vi "Check CSM Modules Exist Or Not.vi"(8 "error in":errorcluster, 11 "CSM names in":string[](array[string])) -> (0 "error out":errorcluster, 2 "Debug string":string, 3 "All Modules Exist?":bool)   [LabVIEW 2017]
uses:
  src/user.lib/_NEVSTOP/Communicable State Machine(CSM)/Communicable State Machine.lvlib
  src/user.lib/_NEVSTOP/Communicable State Machine(CSM)/_Shared/CSM Shared.lvlib
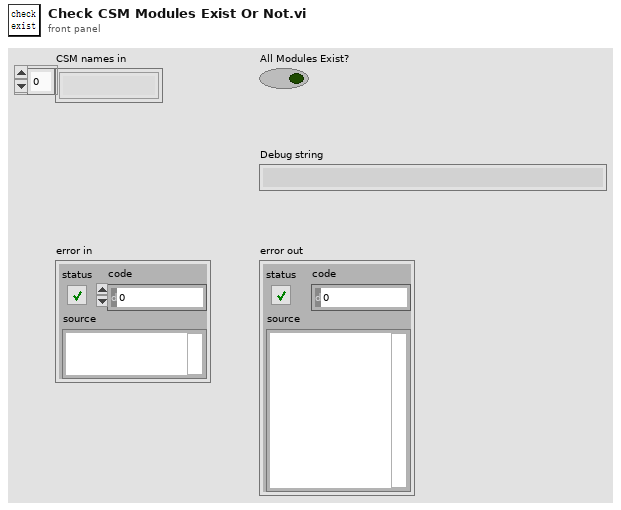
[diagram p1: front panel]
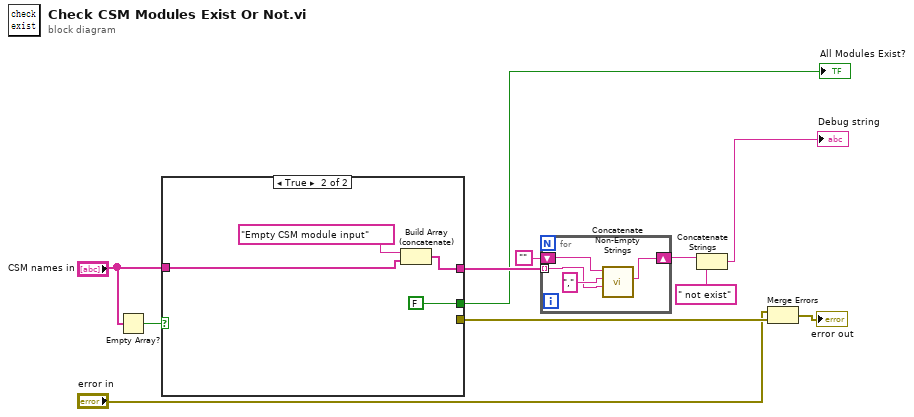
[diagram p0: block diagram]
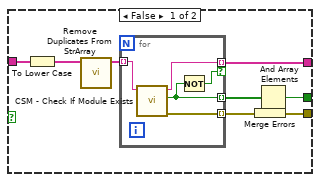
[diagram p2: hidden frame]
diagram:
  n1 = Empty Array?(array="CSM names in") -> (empty?=w2:bool)
  n2 = case shown="True" w2 {
    tunnel: "CSM names in" -> [w18 w26]
    tunnel: [w16 w25] -> w7
    tunnel: [w15 _] -> w6
    tunnel: [w13 FALSE] -> w5
    frame False {
      n3 = To Lower Case(string=w18) -> (all lower case string=w19:string[])
      n4 = call "Remove Duplicates From StrArray.vi"("StrArray In"=w19) -> ("StrArray"=w17:string[])  [unwired: 9 in, 1 out]
      n5 = for {
        tunnel: [w22] -> w12 mode=indexing
        tunnel: [w24] -> w14 mode=indexing
        tunnel: [w23] -> w16 mode=indexing if=w21
        tunnel: w17 -> [w20] mode=indexing
        n6 = call "CSM - Check If Module Exists.vi"("CSM Name"=w20) -> ("error out"=w24:errorcluster, "Exist?"=w22:bool, "CSM Name (Dup)"=w23:string)  [unwired: 8 in]
        n7 = Not(x=w22) -> (.not. x?=w21:bool)
      }
      n8 = Merge Errors(w14) -> (w15:errorcluster)
      n9 = And Array Elements(Boolean array=w12) -> (logical AND=w13:bool)
    }
    frame True {
      n10 = Build Array (concatenate)("Empty CSM module input", w26) -> (w25:string[])
    }
  }
  "All Modules Exist?" <- w5
  n11 = for {
    tunnel: w7 -> [w29] mode=indexing
    shift-right: [w32] -> w9
    shift-left: "" -> [w31]
    n12 = call "Concatenate Non-Empty Strings.vi"("String2"=w29, "Seperator(Carriage Return)"=",", "String1"=w31) -> ("Result String"=w32:string)  [unwired: 5 in]
  }
  n13 = Concatenate Strings(w9, " not exist" ("string")) -> (→"Debug string":string)
  n14 = Merge Errors("error in", w6) -> (→"error out":errorcluster)
